vi "Facade.vi"(0 "Data In":T6, 2 "Display State In":T3={"Title"="", "Explanation"="", "Mode"=enum."myRIO-1900"}, 3 "Container State":T5) -> (6 "Data Out":T6, 7 "Display State Out":T3={"Title"="", "Explanation"="", "Mode"=enum."myRIO-1900"}, 8 "Action":T2)   [LabVIEW 2021, in "myRIO Device Button.xctl"]
uses:
  <vilib>/myRIO/Common/Instrument Driver Framework/Utilities/xctls/myRIO Device Button/myRIO Device Button.xctl
  <vilib>/myRIO/Common/Instrument Driver Framework/Utilities/xctls/myRIO Device Button/Data.ctl
  <vilib>/_xctls/Container State.ctl
  <vilib>/myRIO/Common/Instrument Driver Framework/Utilities/xctls/myRIO Device Button/State.ctl
  <vilib>/myRIO/Common/Instrument Driver Framework/Utilities/typedefs/Hardware Version Enum.ctl
  <vilib>/_xctls/Action.ctl
  <vilib>/myRIO/Common/Instrument Driver Framework/Utilities/xctls/myRIO Device Button/typedefs/Target Image.ctl
  <vilib>/Utility/miscctls.llb/LVPositionTypeDef.ctl
  <vilib>/Utility/miscctls.llb/LVBoundsTypeDef.ctl
  <vilib>/_xctls/XControlSupport.lvlib
panel:
  out "Button Square":picture
  out "Device Image Ring":T1
  out "Explanation":string
  out "Title":string
  out "Background":picture
types:
  T1 = typedef "myRIO Device Button.xctl/Target Image.ctl" = u32
  T2 = typedef "XControlSupport.lvlib/Action.ctl" = cluster{"Data Changed?":bool, "State Changed?":bool, "Action Name":string}
  T3 = typedef "myRIO Device Button.xctl/State.ctl" = cluster{"Title":string, "Explanation":string, "Mode":T4}
  T4 = typedef "Hardware Version Enum.ctl" = enum16{"Unknown", "myRIO-1900", "myRIO-1950", "roboRIO", "NI ELVIS RIO CM", "ELVIS III"}
  T5 = typedef "XControlSupport.lvlib/Container State.ctl" = cluster{"Indicator?":bool, "Run Mode?":bool, " Refnum":refnum<vi>}
  T6 = typedef "myRIO Device Button.xctl/Data.ctl" = bool
  T7 = typedef "LVPositionTypeDef.ctl" = cluster{"Left":i32, "Top":i32}
  T8 = typedef "LVBoundsTypeDef.ctl" = cluster{"Width":u32, "Height":u32}
  T9 = typedef "LVFontTypeDef.ctl" = cluster{"Font Name":string, "Size":u16, "Bold":bool, "Italic":bool, "Underline":bool, "Strikeout":bool, "Color":u32}
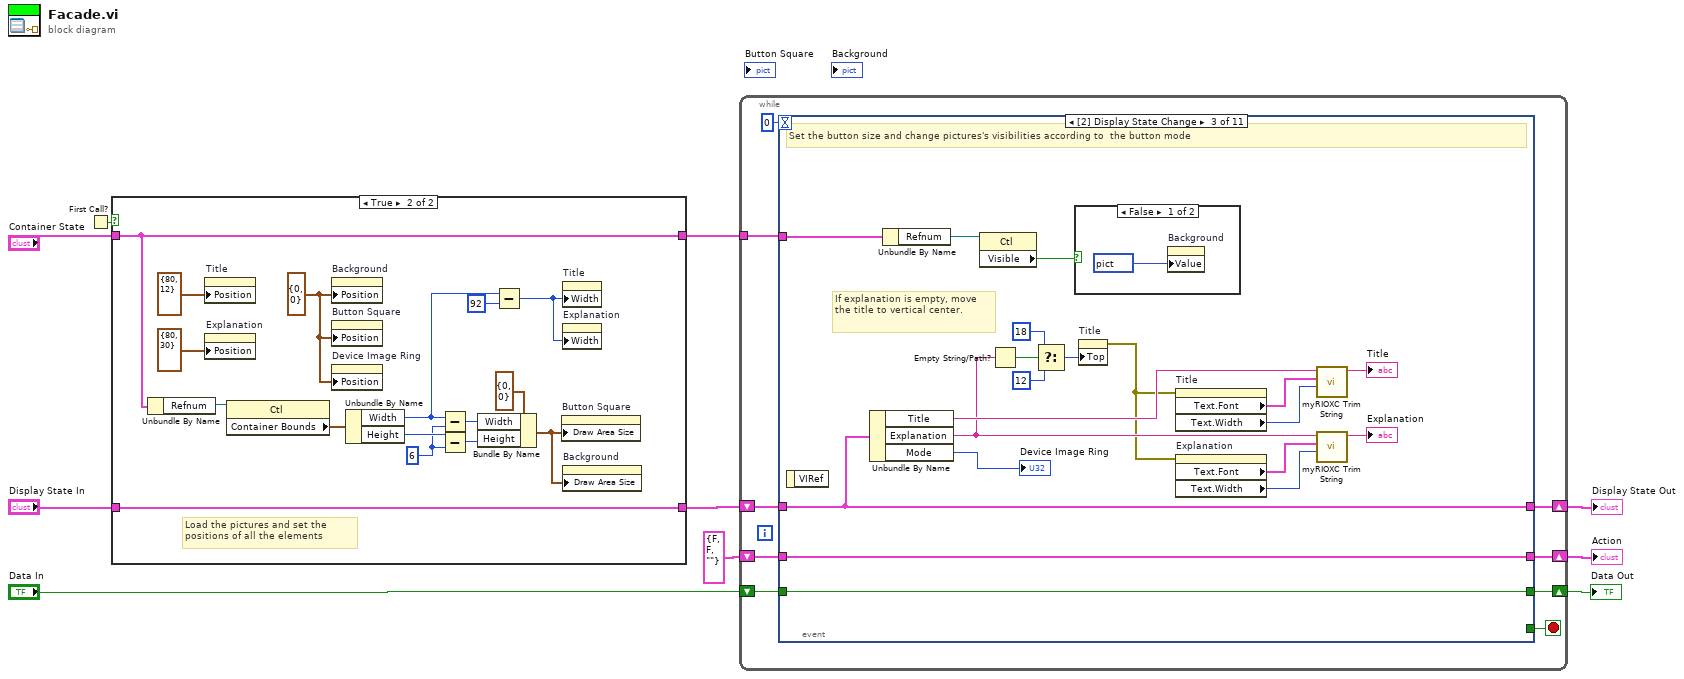
[diagram p0: block diagram]
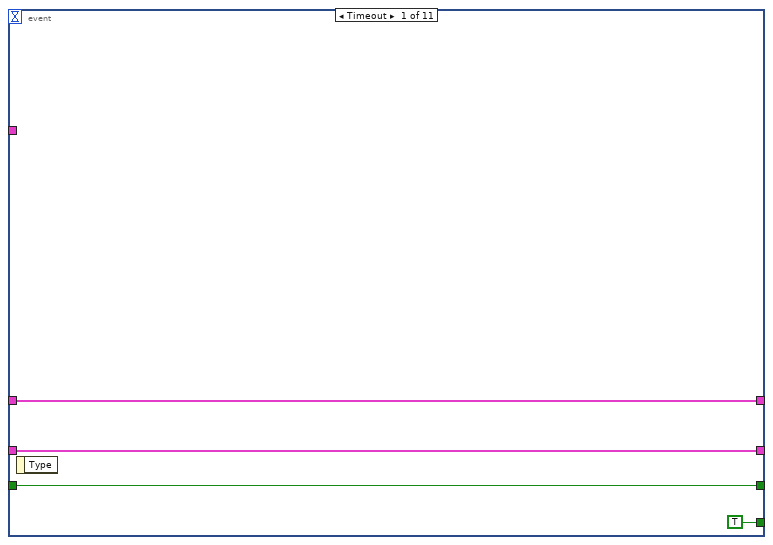
[diagram p3: hidden frame]
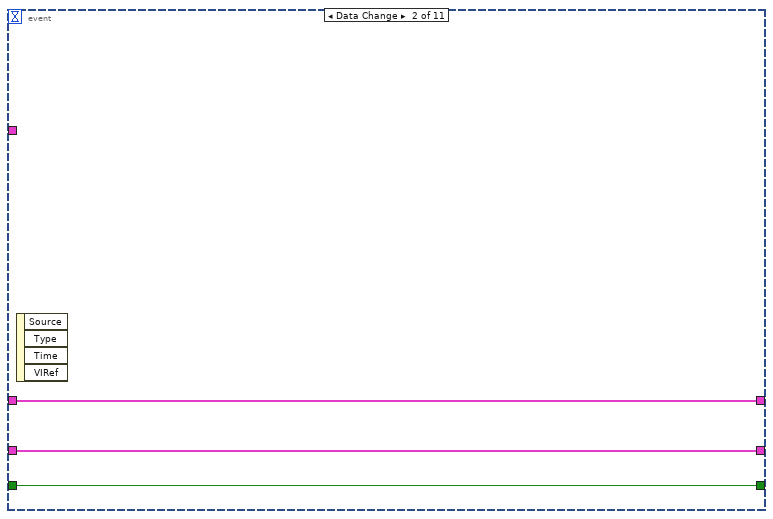
[diagram p4: hidden frame]
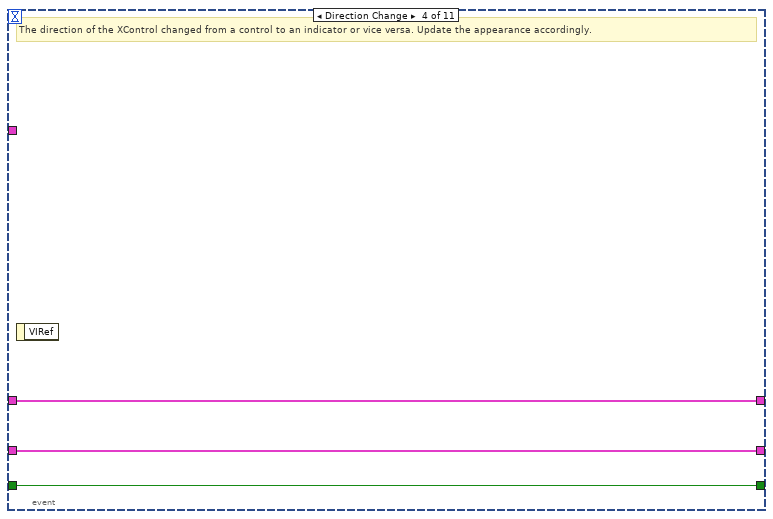
[diagram p6: hidden frame]
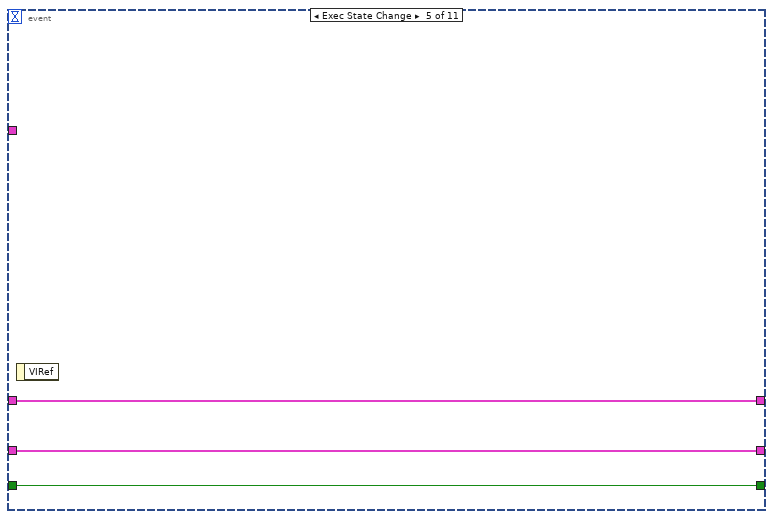
[diagram p7: hidden frame]
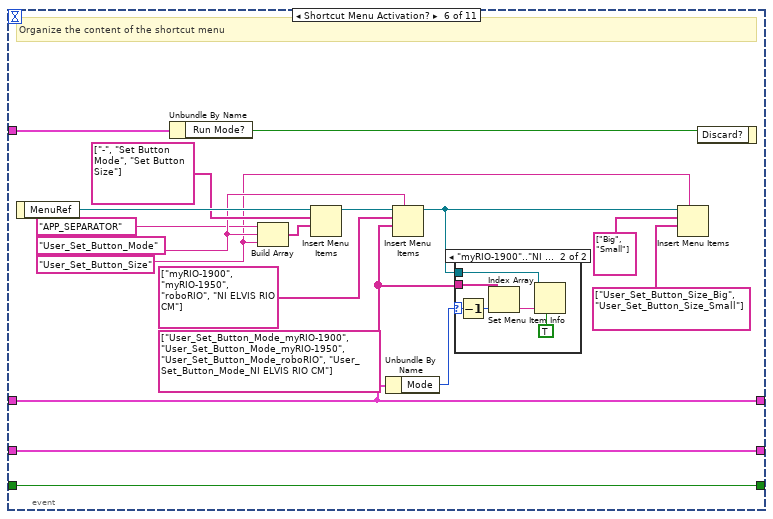
[diagram p8: hidden frame]
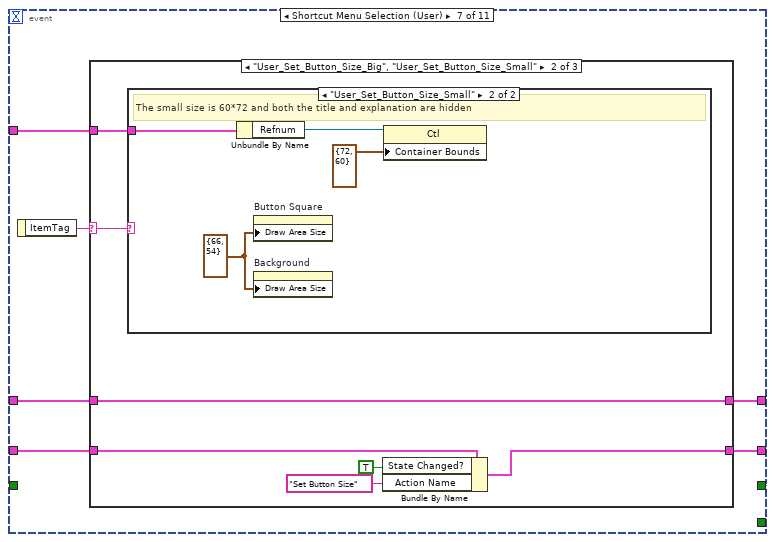
[diagram p10: hidden frame]
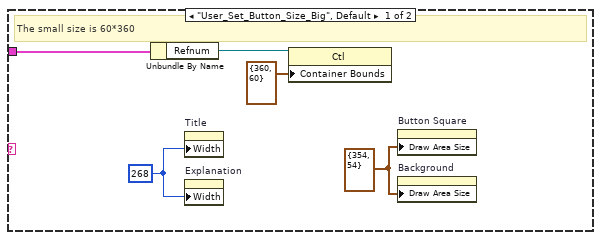
[diagram p12: hidden frame]
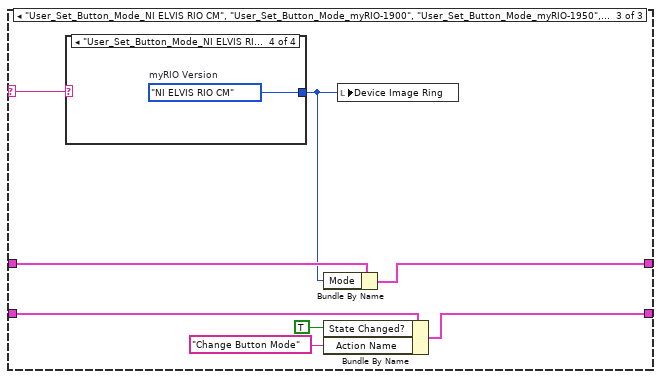
[diagram p13: hidden frame]
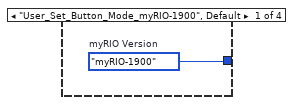
[diagram p14: hidden frame]
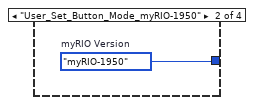
[diagram p15: hidden frame]
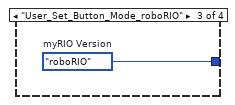
[diagram p16: hidden frame]
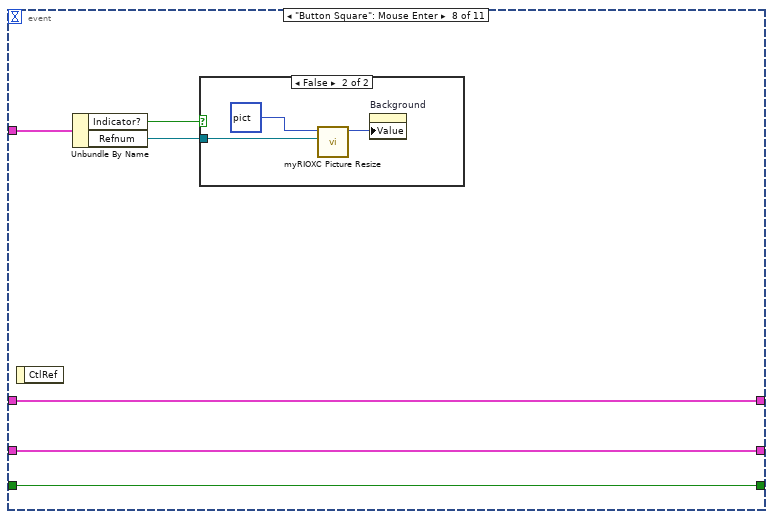
[diagram p17: hidden frame]
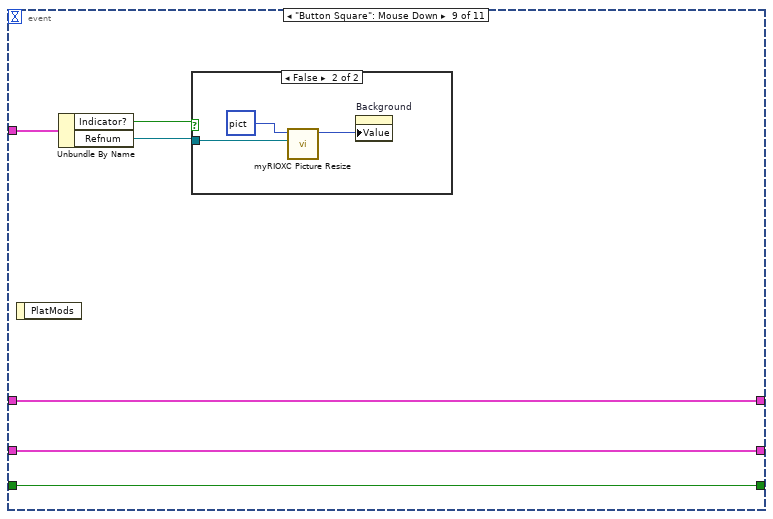
[diagram p19: hidden frame]
diagram:
  n1 = First Call?() -> (First Call?: T/F=w6:bool)
  n2 = case shown="True" w6 {
    tunnel: "Display State In" -> [w12 w28]
    tunnel: [w12 w28] -> w4
    tunnel: "Container State" -> [w11 w17]
    tunnel: [w11 w17] -> w2
    frame False {
    }
    frame True {
      w22 = u32 6 ("y")
      w16 = T7 {"Left"=0, "Top"=0} ("Position")
      # "Load the pictures and set the positions of all the elements"
      n3 = Unbundle By Name(w17) -> ("Refnum"=w13:refnum<vi>)
      n4 = property on="Title" class="Str"("Position"=T7 {"Left"=80, "Top"=12}) -> ()  [unwired: 2 in, 2 out]
      n5 = property on="Explanation" class="Str"("Position"=T7 {"Left"=80, "Top"=30}) -> ()  [unwired: 2 in, 2 out]
      n6 = property class="Ctl"(reference=w13) -> ("Container Bounds"=w27:T8)  [unwired: 1 in, 2 out]
      n7 = property on="Background" class="Pict"("Position"=w16) -> ()  [unwired: 2 in, 2 out]
      n8 = property on="Button Square" class="Pict"("Position"=w16) -> ()  [unwired: 2 in, 2 out]
      n9 = property on="Device Image Ring" class="Ring (strict)"("Position"=w16) -> ()  [unwired: 2 in, 2 out]
      n10 = Unbundle By Name(w27) -> ("Width"=w18:u32, "Height"=w23:u32)
      n11 = Subtract(x=w18, y=w22) -> (x-y=w26:u32)
      n12 = Subtract(x=w23, y=w22) -> (x-y=w25:u32)
      n13 = Bundle By Name(cluster=T8 {"Width"=0, "Height"=0} ("Draw Area Size"), "Width"=w26, "Height"=w25) -> (w21:T8)
      n14 = Subtract(x=w18, y=u32 92) -> (x-y=w19:u32)
      n15 = property on="Button Square" class="Pict"("Draw Area Size"=w21) -> ()  [unwired: 2 in, 2 out]
      n16 = property on="Title" class="Str"("Width"=w19) -> ()  [unwired: 2 in, 2 out]
      n17 = property on="Explanation" class="Str"("Width"=w19) -> ()  [unwired: 2 in, 2 out]
      n18 = property on="Background" class="Pict"("Draw Area Size"=w21) -> ()  [unwired: 2 in, 2 out]
    }
  }
  n19 = while {
    shift-right: [w36] -> w9
    shift-left: w4 -> [w37]
    tunnel: w2 -> [w33]
    shift-right: [w31] -> w10
    shift-left: "Data In" -> [w32]
    shift-right: [w29] -> w8
    shift-left: T2 {"Data Changed?"=FALSE, "State Changed?"=FALSE, "Action Name"=""} ("Action") -> [w30]
    stop <- w35 stop-if-true
    n20 = event shown="[2] Display State Change" {
      selector: _ -> [_ _ _ _ _ _ _ _ _ _ _]
      dyn-events: _ -> [_ _ _ _ _ _ _ _ _ _ _]
      timeout: 0 -> [_ _ _ _ _ _ _ _ _ _ _]
      tunnel: w37 -> [w38 w43 w61 w68 w71 w81 w100 w138 w147 w155 w164]
      tunnel: [w38 w43 w61 w68 w71 w81 w97 w138 w147 w155 w164] -> w36
      tunnel: [TRUE _ _ _ _ _ _ _ _ _ _] -> w35
      tunnel: w33 -> [_ _ w47 _ _ w86 w96 w135 w146 w152 w163]
      tunnel: w32 -> [w39 w44 w64 w67 w70 w89 w102 w137 w142 w154 w158]
      tunnel: [w39 w44 w64 w67 w70 w89 w102 w137 w142 w154 w157] -> w31
      tunnel: [w40 w42 w63 w66 w69 w88 w98 w136 w143 w153 w159] -> w29
      tunnel: w30 -> [w40 w42 w63 w66 w69 w88 w99 w136 w143 w153 w160]
      event Timeout {
        n21 = event-data() -> ()  [unwired: 1 in, 1 out]
      }
      event Data Change {
        n22 = event-data() -> ()  [unwired: 1 in, 4 out]
      }
      event Display State Change {
        # "If explanation is empty, move the title to vertical center."
        # "Set the button size and change pictures's visibilities according to  the button mode"
        n23 = event-data() -> ()  [unwired: 1 in, 1 out]
        n24 = Unbundle By Name(w61) -> ("Title"=w60:string, "Explanation"=w59:string, "Mode"=→"Device Image Ring":T4)
        n25 = Unbundle By Name(w47) -> ("Refnum"=w46:refnum<vi>)
        n26 = property class="Ctl"(reference=w46) -> ("Visible"=w45:bool)  [unwired: 1 in, 2 out]
        n27 = Empty String/Path?(string/path=w59) -> (empty?=w56:bool)
        n28 = Select(t=18 ("Top"), s=w56, f=12 ("Top")) -> (s? t:f=w62:i32)
        n29 = case shown="False" w45 {
          frame False {
            n30 = property on="Background" class="Pict"("Value"=picture bytes[56344] ("Mouse Leave Background")) -> ()  [unwired: 2 in, 2 out]
          }
          frame True {
          }
        }
        n31 = property on="Title" class="Str"("Top"=w62) -> (error out=w48:errorcluster)  [unwired: 2 in, 1 out]
        n32 = property on="Title" class="Str"(error in=w48) -> ("Text.Font"=w52:T9, "Text.Width"=w49:u32)  [unwired: 1 in, 2 out]
        n33 = property on="Explanation" class="Str"(error in=w48) -> ("Text.Font"=w51:T9, "Text.Width"=w50:u32)  [unwired: 1 in, 2 out]
        n34 = call <vilib>:"myRIOXC Trim String.vi"("Max Length"=w49, "Text Font"=w52, "Input Text"=w60) -> ("Output Text"=→"Title":string)  [unwired: 8 in]
        n35 = call <vilib>:"myRIOXC Trim String.vi"("Max Length"=w50, "Text Font"=w51, "Input Text"=w59) -> ("Output Text"=→"Explanation":string)  [unwired: 8 in]
      }
      event Direction Change {
        # "The direction of the XControl changed from a control to an indicator or vice versa. Update the appearance accordingly."
        n36 = event-data() -> ()  [unwired: 1 in, 1 out]
      }
      event Exec State Change {
        n37 = event-data() -> ()  [unwired: 1 in, 1 out]
      }
      event Shortcut Menu Activation? {
        w75 = "User_Set_Button_Size"
        w73 = string[] ["User_Set_Button_Mode_myRIO-1900", "User_Set_Button_Mode_myRIO-1950", "User_Set_Button_Mode_roboRIO", "User_Set_Button_Mode_NI ELVIS RIO CM"]
        w79 = "User_Set_Button_Mode"
        # "Organize the content of the shortcut menu"
        n38 = event-data() -> ("MenuRef"=w87:refnum<k9>)  [unwired: 1 in]
        n39 = Unbundle By Name(w86) -> ("Run Mode?"=w85:bool)
        n40 = Build Array("APP_SEPARATOR", w79, w75) -> (w82:string[])
        n41 = Insert Menu Items(7:w82, 8:string[] ["-", "Set Button Mode", "Set Button Size"], 9:w87) -> (3:w83:refnum<k9>)  [unwired: 3 in, 2 out]
        n42 = Unbundle By Name(w81) -> ("Mode"=w74:T4)
        n43 = Insert Menu Items(5:w79, 7:w73, 8:string[] ["myRIO-1900", "myRIO-1950", "roboRIO", "NI ELVIS RIO CM"], 9:w83) -> (3:w72:refnum<k9>)  [unwired: 2 in, 2 out]
        n44 = case shown="\"myRIO-1900\"..\"NI ELVIS RIO CM\"" w74 {
          selector: w74 -> [_ w91]
          tunnel: w73 -> [_ w93]
          tunnel: w72 -> [_ w90]
          frame "Unknown", Default {
          }
          frame "myRIO-1900".."NI ELVIS RIO CM" {
            n45 = Decrement(x=w91) -> (x-1=w92:T4)
            n46 = Index Array(array=w93, index=w92) -> (element=w94:string)
            n47 = Set Menu Item Info(6:TRUE, 7:w94, 11:w90) -> ()  [unwired: 4 in, 2 out]
          }
        }
        n48 = Insert Menu Items(5:w75, 7:string[] ["User_Set_Button_Size_Big", "User_Set_Button_Size_Small"], 8:string[] ["Big", "Small"], 9:w72) -> ()  [unwired: 2 in, 3 out]
        n49 = event-data("Discard?"=w85) -> ()  [unwired: 1 in, 1 out]
      }
      event Shortcut Menu Selection (User) {
        n50 = event-data() -> ("ItemTag"=w101:string)  [unwired: 1 in]
        n51 = case shown="\"User_Set_Button_Size_Big\", \"User_Set_Button_Size_Small\"" w101 {
          selector: w101 -> [_ w110 w128]
          tunnel: [w104 w106 w122] -> w97
          tunnel: w100 -> [w104 w106 w123]
          tunnel: w99 -> [w103 w108 w127]
          tunnel: [w103 w107 w125] -> w98
          tunnel: w96 -> [_ w111 _]
          frame Default {
          }
          frame "User_Set_Button_Size_Big", "User_Set_Button_Size_Small" {
            n52 = case shown="\"User_Set_Button_Size_Small\"" w110 {
              tunnel: w111 -> [w116 w118]
              frame "User_Set_Button_Size_Big", Default {
                w112 = u32 268 ("Size:Width")
                w113 = T8 {"Width"=354, "Height"=54} ("Draw Area Size")
                # "The small size is 60*360"
                n53 = Unbundle By Name(w116) -> ("Refnum"=w114:refnum<vi>)
                n54 = property on="Title" class="Str"("Width"=w112) -> ()  [unwired: 2 in, 2 out]
                n55 = property on="Explanation" class="Str"("Width"=w112) -> ()  [unwired: 2 in, 2 out]
                n56 = property class="Ctl"(reference=w114, "Container Bounds"=T8 {"Width"=360, "Height"=60} ("XControl:Container Bounds")) -> ()  [unwired: 1 in, 2 out]
                n57 = property on="Button Square" class="Pict"("Draw Area Size"=w113) -> ()  [unwired: 2 in, 2 out]
                n58 = property on="Background" class="Pict"("Draw Area Size"=w113) -> ()  [unwired: 2 in, 2 out]
              }
              frame "User_Set_Button_Size_Small" {
                w117 = T8 {"Width"=66, "Height"=54} ("Draw Area Size")
                # "The small size is 60*72 and both the title and explanation are hidden"
                n59 = Unbundle By Name(w118) -> ("Refnum"=w120:refnum<vi>)
                n60 = property on="Button Square" class="Pict"("Draw Area Size"=w117) -> ()  [unwired: 2 in, 2 out]
                n61 = property on="Background" class="Pict"("Draw Area Size"=w117) -> ()  [unwired: 2 in, 2 out]
                n62 = property class="Ctl"(reference=w120, "Container Bounds"=T8 {"Width"=72, "Height"=60} ("XControl:Container Bounds")) -> ()  [unwired: 1 in, 2 out]
              }
            }
            n63 = Bundle By Name(cluster=w108, "State Changed?"=TRUE, "Action Name"="Set Button Size") -> (w107:T2)
          }
          frame "User_Set_Button_Mode_NI ELVIS RIO CM", "User_Set_Button_Mode_myRIO-1900", "User_Set_Button_Mode_myRIO-1950", "User_Set_Button_Mode_roboRIO" {
            n64 = case shown="\"User_Set_Button_Mode_NI ELVIS RIO CM\"" w128 {
              tunnel: [w129 w130 w131 w132] -> w121
              frame "User_Set_Button_Mode_myRIO-1900", Default {
                w129 = Hardware_Version_Enum."myRIO-1900"  # myRIO Version
              }
              frame "User_Set_Button_Mode_myRIO-1950" {
                w130 = Hardware_Version_Enum."myRIO-1950"  # myRIO Version
              }
              frame "User_Set_Button_Mode_roboRIO" {
                w131 = Hardware_Version_Enum."roboRIO"  # myRIO Version
              }
              frame "User_Set_Button_Mode_NI ELVIS RIO CM" {
                w132 = Hardware_Version_Enum."NI ELVIS RIO CM"  # myRIO Version
              }
            }
            n65 = Bundle By Name(cluster=w123, "Mode"=w121) -> (w122:T3)
            n66 = Bundle By Name(cluster=w127, "State Changed?"=TRUE, "Action Name"="Change Button Mode") -> (w125:T2)
            n67 = local write "Device Image Ring"(w121) -> ()
          }
        }
      }
      event "Button Square": Mouse Enter {
        n68 = event-data() -> ()  [unwired: 1 in, 1 out]
        n69 = Unbundle By Name(w135) -> ("Indicator?"=w134:bool, "Refnum"=w133:refnum<vi>)
        n70 = case shown="False" w134 {
          tunnel: w133 -> [_ w140]
          frame True {
          }
          frame False {
            n71 = call <vilib>:"myRIOXC Picture Resize.vi"("XCtrl Reference"=w140, "picture"=picture bytes[56344] ("Mouse Enter Background")) -> ("new picture"=w139:picture)  [unwired: 9 in]
            n72 = property on="Background" class="Pict"("Value"=w139) -> ()  [unwired: 2 in, 2 out]
          }
        }
      }
      event "Button Square": Mouse Down {
        n73 = event-data() -> ()  [unwired: 1 in, 1 out]
        n74 = Unbundle By Name(w146) -> ("Indicator?"=w144:bool, "Refnum"=w145:refnum<vi>)
        n75 = case shown="False" w144 {
          tunnel: w145 -> [_ w149]
          frame True {
          }
          frame False {
            n76 = call <vilib>:"myRIOXC Picture Resize.vi"("XCtrl Reference"=w149, "picture"=picture bytes[56344] ("Mouse Down Background")) -> ("new picture"=w148:picture)  [unwired: 9 in]
            n77 = property on="Background" class="Pict"("Value"=w148) -> ()  [unwired: 2 in, 2 out]
          }
        }
      }
      event "Button Square": Mouse Leave {
        n78 = event-data() -> ()  [unwired: 1 in, 1 out]
        n79 = Unbundle By Name(w152) -> ("Indicator?"=w151:bool)
        n80 = case shown="False" w151 {
          frame True {
          }
          frame False {
            n81 = property on="Background" class="Pict"("Value"=picture bytes[56344] ("Mouse Leave Background")) -> ()  [unwired: 2 in, 2 out]
          }
        }
      }
      event "Button Square": Mouse Up {
        n82 = event-data() -> ()  [unwired: 1 in, 1 out]
        n83 = Unbundle By Name(w163) -> ("Indicator?"=w162:bool, "Refnum"=w161:refnum<vi>)
        n84 = case shown="False" w162 {
          tunnel: w161 -> [_ w168]
          tunnel: w160 -> [w165 w170]
          tunnel: [w165 w169] -> w159
          frame True {
          }
          frame False {
            n85 = Bundle By Name(cluster=w170, "Data Changed?"=TRUE) -> (w169:T2)
            n86 = call <vilib>:"myRIOXC Picture Resize.vi"("XCtrl Reference"=w168, "picture"=picture bytes[56344] ("Mouse Enter Background")) -> ("new picture"=w167:picture)  [unwired: 9 in]
            n87 = property on="Background" class="Pict"("Value"=w167) -> ()  [unwired: 2 in, 2 out]
          }
        }
        n88 = Not(x=w158) -> (.not. x?=w157:T6)
      }
    }
  }
  "Display State Out" <- w9
  "Data Out" <- w10
  "Action" <- w8
